vi "WSVCAP SHL Host TL I2C Write.vi"(0 "C Data Out":u8[][](array[numeric]) format="%.0x", 1 "Socket Mask [U64]":u64 format="%012x", 11 "error in":errorcluster, 12 "Sub Address":u8=20, 13 "Log (T)":bool=TRUE, 14 "FPGA":T1) -> (15 "error out":errorcluster)   [LabVIEW 2017]
uses:
  Type Defs/WSVCAP SHL FPGA Enum.ctl
  Type Defs/WSVCAP SHL Function Enum.ctl
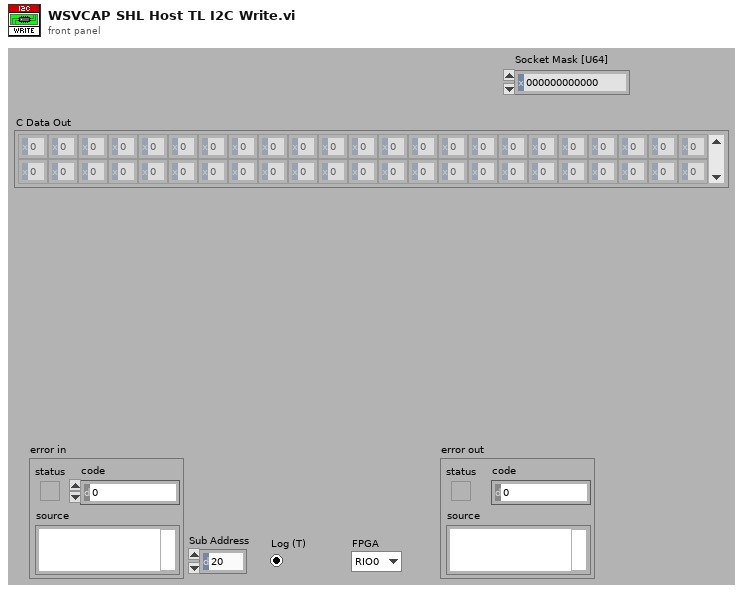
[diagram p1: front panel]
types:
  T1 = typedef "WSVCAP SHL FPGA Enum.ctl" = enum16{"RIO0", "RIO1"}
  T2 = typedef "WSVCAP SHL Function Enum.ctl" = enum16{"Initialize", "Configure I2C", "Configure RFFE", "Write I2C", "Read I2C", "Write RFFE", "Read RFFE", "Start RFFE Cycle", "Stop RFFE Cycle", "Get Status", "Close"}
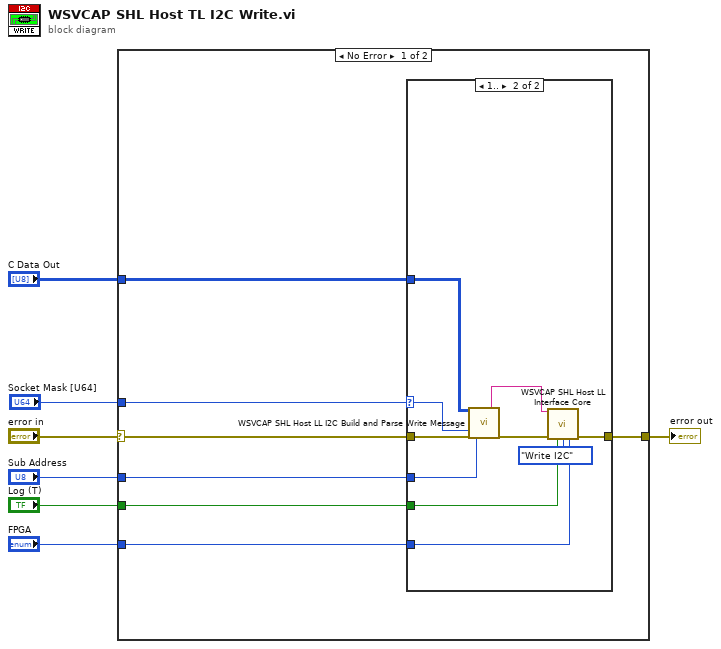
[diagram p0: block diagram]
diagram:
  n1 = case shown="No Error" "error in" {
    selector: "error in" -> [w13 w26]
    tunnel: [w14 w26] -> w7
    tunnel: "C Data Out" -> [w8 _]
    tunnel: "Sub Address" -> [w10 _]
    tunnel: "Socket Mask [U64]" -> [w12 _]
    tunnel: "Log (T)" -> [w11 _]
    tunnel: "FPGA" -> [w9 _]
    frame No Error {
      n2 = case shown="1.." w12 {
        selector: w12 -> [_ w20]
        tunnel: [w15 w24] -> w14
        tunnel: w13 -> [w15 w23]
        tunnel: w11 -> [_ w19]
        tunnel: w8 -> [_ w18]
        tunnel: w10 -> [_ w17]
        tunnel: w9 -> [_ w16]
        frame ..0 {
        }
        frame 1.. {
          n3 = call "WSVCAP SHL Host LL I2C Build and Parse Write Message.vi"("C Write Data In [DUT Ordered]"=w18, "Socket Mask [U64] In"=w20, "error in"=w23, "Sub Address In"=w17) -> ("Message Out"=w21:string, "error out"=w22:errorcluster)  [unwired: 10 in, 4 out]
          n4 = call "WSVCAP SHL Host LL Interface Core.vi"("Message In"=w21, "error in"=w22, "Log (T)"=w19, "Function"=WSVCAP_SHL_Function_Enum."Write I2C", "FPGA"=w16) -> ("error out"=w24:errorcluster)  [unwired: 8 in, 2 out]
        }
      }
    }
    frame Error {
    }
  }
  "error out" <- w7
